vi "EnableMotors.vi"(8 "error in (no error)":errorcluster, 9 "Link 2 Demand":dbl, 11 "Link 1 Demand":dbl) -> (0 "error out":errorcluster, 2 "Enable motor 2":bool, 3 "Enable motor 1":bool)   [LabVIEW 2017, in "lowLevelController.lvlib"]
doc: "This VI enables and disables the motors, depending on whether the absolute value of demand is above 0\n\nThe equates to activating and deactivating relays via the FPGA."
uses:
  lowLevelController.lvlib
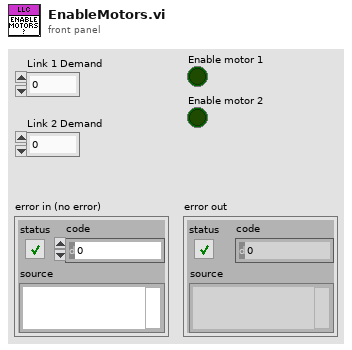
[diagram p1: front panel]
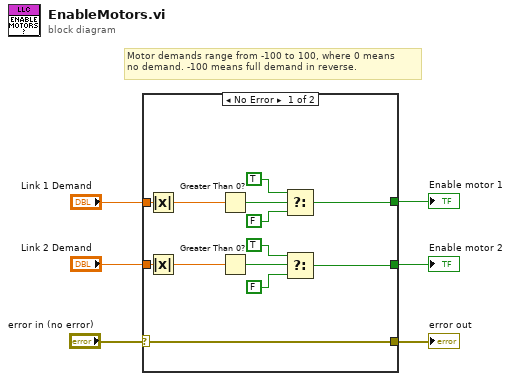
[diagram p0: block diagram]
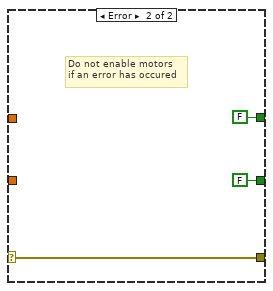
[diagram p2: hidden frame]
diagram:
  # "Motor demands range from -100 to 100, where 0 means\nno demand. -100 means full demand in reverse."
  n1 = case shown="No Error" "error in (no error)" {
    selector: "error in (no error)" -> [w9 w22]
    tunnel: "Link 1 Demand" -> [w19 _]
    tunnel: "Link 2 Demand" -> [w18 _]
    tunnel: [w11 FALSE] -> w4
    tunnel: [w10 FALSE] -> w3
    tunnel: [w9 w22] -> w1
    frame No Error {
      n2 = Absolute Value(x=w19) -> (abs(x)=w8:dbl)
      n3 = Absolute Value(x=w18) -> (abs(x)=w7:dbl)
      n4 = Greater Than 0?(x=w8) -> (x > 0?=w17:bool)
      n5 = Greater Than 0?(x=w7) -> (x > 0?=w16:bool)
      n6 = Select(t=TRUE, s=w17, f=FALSE) -> (s? t:f=w11:bool)
      n7 = Select(t=TRUE, s=w16, f=FALSE) -> (s? t:f=w10:bool)
    }
    frame Error {
      # "Do not enable motors\nif an error has occured"
    }
  }
  "error out" <- w1
  "Enable motor 1" <- w4
  "Enable motor 2" <- w3
